vi "LVClass_DataClient GetNumberOfServerData.vi"(0 "DataClient in":refnum<class "DataClient.lvclass">, 11 "error in (no error)":errorcluster) -> (4 "DataClient out":refnum<class "DataClient.lvclass">, 10 "Number of data":i32, 15 "error out":errorcluster)   [LabVIEW 2020, in "DataClient.lvclass"]
doc: "Slopes getter.\n\n<B>clientIn</B> : Client object.\n<B>clientOut</B> : Client object.\n<B>data_number</B> : Number of data server can send (useful to allocate data names and types\n arrays)."
uses:
  DataClient.lvclass
  DataClient.lvclass/DataClient.ctl
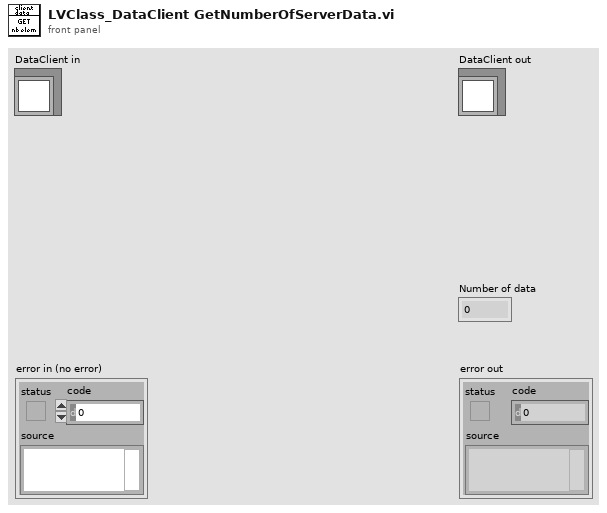
[diagram p1: front panel]
types:
  T1 = typedef "ClassID.ctl" = i64
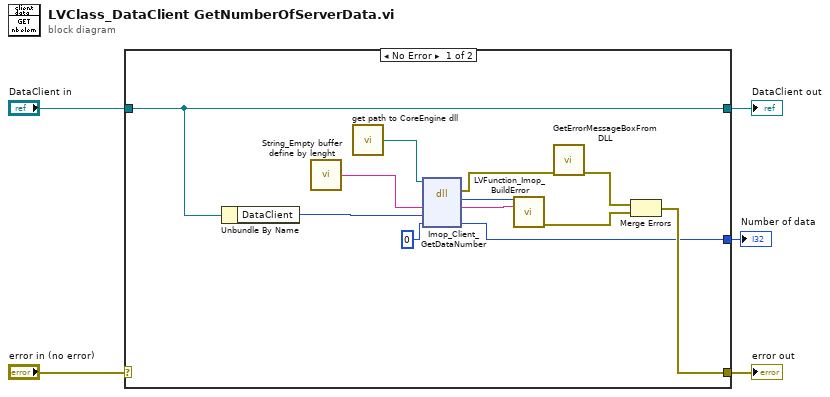
[diagram p0: block diagram]
diagram:
  n1 = case shown="No Error" "error in (no error)" {
    selector: "error in (no error)" -> [_ w19]
    tunnel: [w8 w19] -> w4
    tunnel: [w9 w18] -> w2
    tunnel: "DataClient in" -> [w9 w18]
    tunnel: [w6 _] -> w1
    frame No Error {
      n2 = Unbundle By Name(w9) -> ("DataClient"=w12:T1)
      n3 = call "String_Empty buffer define by lenght.vi"() -> ("Empty buffer"=w15:string)  [unwired: 1 in]
      n4 = call "get path to CoreEngine dll.vi"() -> ("path to wavekit library"=w14:path)  [unwired: 14 in, 1 out]
      n5 = dll-call lib="D:/soft/HASO_v3/SVN_trunk/ImOpCoreEngine4_LV2011/DLLs/c_interface_vc100.dll" fn="Imop_Client_GetDataNumber"(path in=w14, "message"=w15, "client"=w12, "NumberOfData"=0 ("data_id")) -> (error out=w13:errorcluster, "return type"=w17:i32, "message"=w16:string, "NumberOfData"=w6:i32)  [unwired: 3 in, 1 out]
      n6 = call "LVFunction_Imop_BuildError.vi"("code"=w17, "String to Prepend to source (\"\")"=w16) -> ("error out"=w10:errorcluster)  [unwired: 13 in]
      n7 = call "GetErrorMessageBoxFromDLL.vi"("error IN"=w13) -> ("error OUT"=w11:errorcluster)  [unwired: 10 in]
      n8 = Merge Errors(w11, w10) -> (w8:errorcluster)
    }
    frame Error {
    }
  }
  "error out" <- w4
  "DataClient out" <- w2
  "Number of data" <- w1
